vi "GFG refresh all variables.vi"(11 "Variables to refresh":string[](array[string])) -> ()   [LabVIEW 2012, in "GFG library.lvlib"]
uses:
  GFG library.lvlib
panel:
  out "Array":T1(array[cluster])
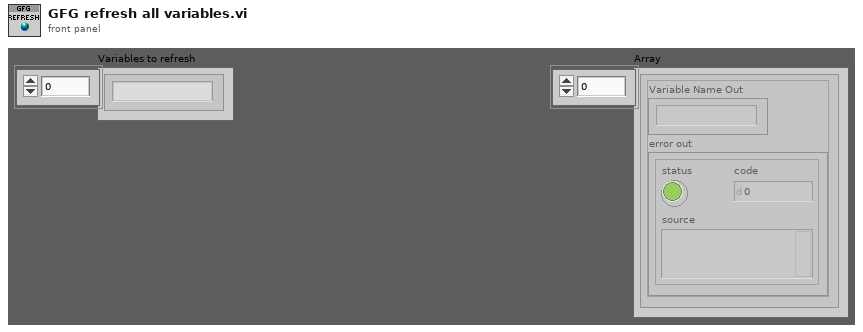
[diagram p1: front panel]
types:
  T1 = cluster{"Variable Name Out":string, "error out":errorcluster}[]
  T2 = cluster{"Variable Name Out":string, "error out":errorcluster}
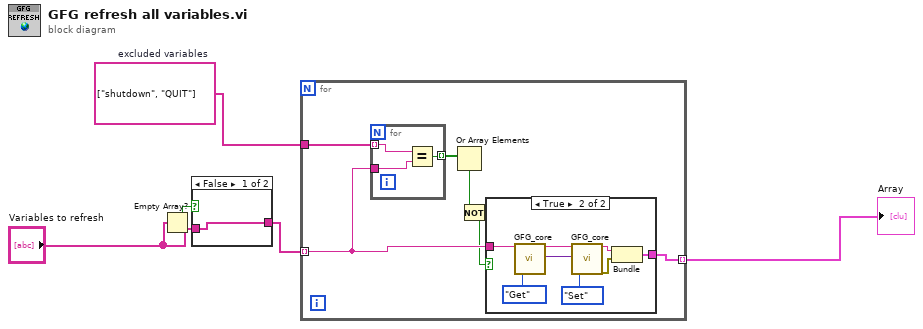
[diagram p0: block diagram]
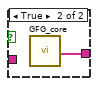
[diagram p2: hidden frame]
diagram:
  w2 = string[] ["shutdown", "QUIT"]  # excluded variables
  n1 = Empty Array?(array="Variables to refresh") -> (empty?=w4:bool)
  n2 = case shown="False" w4 {
    tunnel: [w6 w7] -> w3
    tunnel: "Variables to refresh" -> [w6 _]
    frame False {
    }
    frame True {
      n3 = call "GFG_core.vi"() -> ("All Variable Names Out"=w7:string[])  [unwired: 13 in, 6 out]
    }
  }
  n4 = for {
    tunnel: w3 -> [w11] mode=indexing
    tunnel: [w13] -> w5 mode=indexing
    tunnel: w2 -> [w12]
    n5 = for {
      tunnel: w12 -> [w24] mode=indexing
      tunnel: w11 -> [w23]
      tunnel: [w22] -> w10 mode=indexing
      n6 = Equal?(x=w24, y=w23) -> (x = y?=w22:bool)
    }
    n7 = Or Array Elements(Boolean array=w10) -> (logical OR=w9:bool)
    n8 = Not(x=w9) -> (.not. x?=w8:bool)
    n9 = case shown="True" w8 {
      tunnel: [_ w15] -> w13
      tunnel: w11 -> [_ w14]
      frame False {
      }
      frame True {
        n10 = call "GFG_core.vi"("Variable Name in"=w14, "Action"=enum16{"Init", "Set", "Get"}."Get") -> ("Variable Name Out"=w19:string, "Variant Out"=w18:variant)  [unwired: 11 in, 5 out]
        n11 = call "GFG_core.vi"("Variable Name in"=w19, "Variant in"=w18, "Action"=enum16{"Init", "Set", "Get"}."Set") -> ("Variable Name Out"=w17:string, "error out"=w16:errorcluster)  [unwired: 10 in, 5 out]
        n12 = Bundle("Variable Name Out"=w17, "error out"=w16) -> (w15:T2)  [unwired: 1 in]
      }
    }
  }
  "Array" <- w5
